vi "Car Wash.vi"() -> ()   [LabVIEW 2013]
uses:
  Controls/Car Wash Indicators.ctl
  Controls/Wash Options.ctl
  Controls/Car Wash States.ctl
  Controls/Wash option states.ctl
panel:
  in  "Start":bool
  out "Elapsed Time":dbl format="%0.2f"
  in  "stop":bool
  out "Wash Entry":bool
  in  "Wash Options":T1
  in  "Car Position Slider":u8(slide) max=3 scale=0.0..4.0
  out "Car Wash Indicators":T2
  # "Entry Console"
  # "Car Wash Display"
  # "Car Position Simulation"
  # "Pre-Soak\nH-P Wash\nL-P Wax\nSpot Free Rinse"
  # "Underbody Wash\nBug Remover"
  # "Tire Shine\nAir Dry"
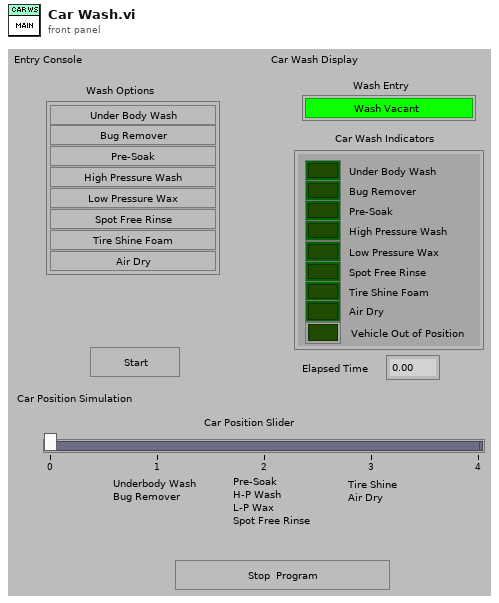
[diagram p1: front panel]
types:
  T1 = typedef "Wash Options.ctl" = cluster{"Underbody Wash":bool, "Bug Remover":bool, "Pre-Soak":bool, "High Pressure Wash":bool, "Low Pressure Wax":bool, "Spot Free Rinse":bool, "Tire Shine Foam":bool, "Air Dry":bool}
  T2 = typedef "Car Wash Indicators.ctl" = cluster{"Under Body Wash":bool, "Bug Remover":bool, "Pre-Soak":bool, "High Pressure Wash":bool, "Low Pressure Wax":bool, "Spot Free Rinse":bool, "Tire Shine Foam":bool, "Air Dry":bool, "Vehicle Out of Position":bool}
  T3 = typedef "Car Wash States.ctl" = enum16{"Initialize", "Start", "Main", "Stop"}
  T4 = enum8{"Enabled", "Disabled", "Disabled and Grayed Out"}
  T5 = typedef "Wash option states.ctl" = enum16{"Under Body Wash", "Bug Remover", "Pre-Soak", "HIgh Pressure Wash", "Low Pessure Wax", "Spot Free rinse", "Tire Shine Foam", "Air Dry", "Exit", "Reset "}
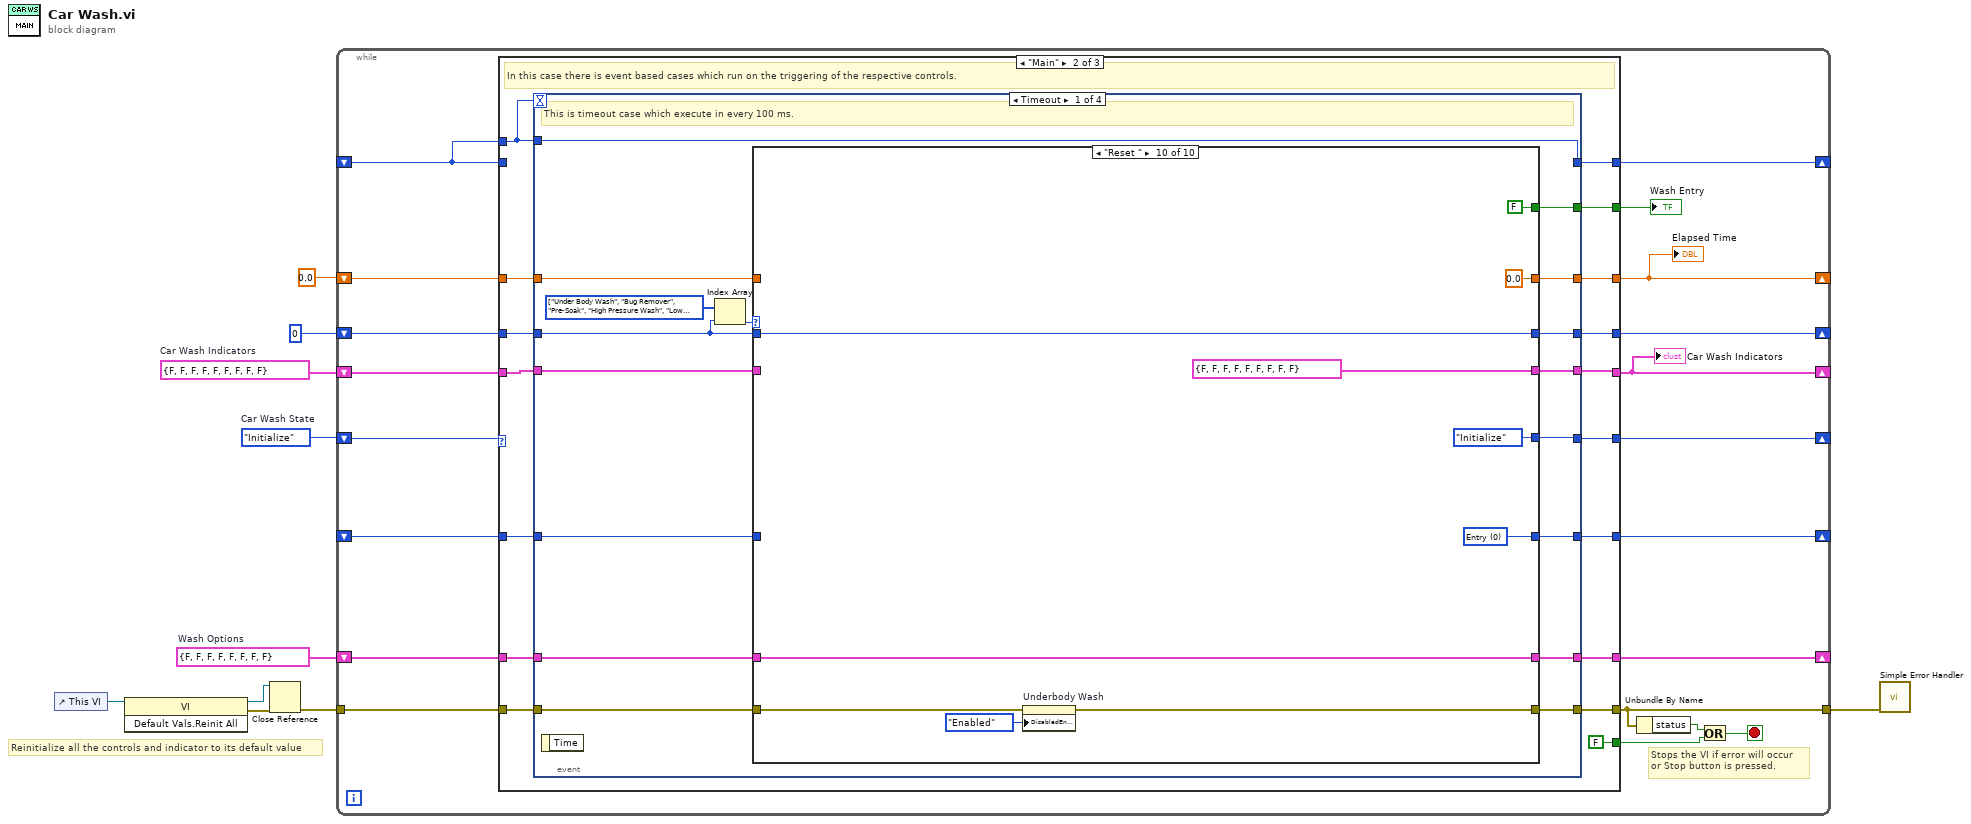
[diagram p0: block diagram]
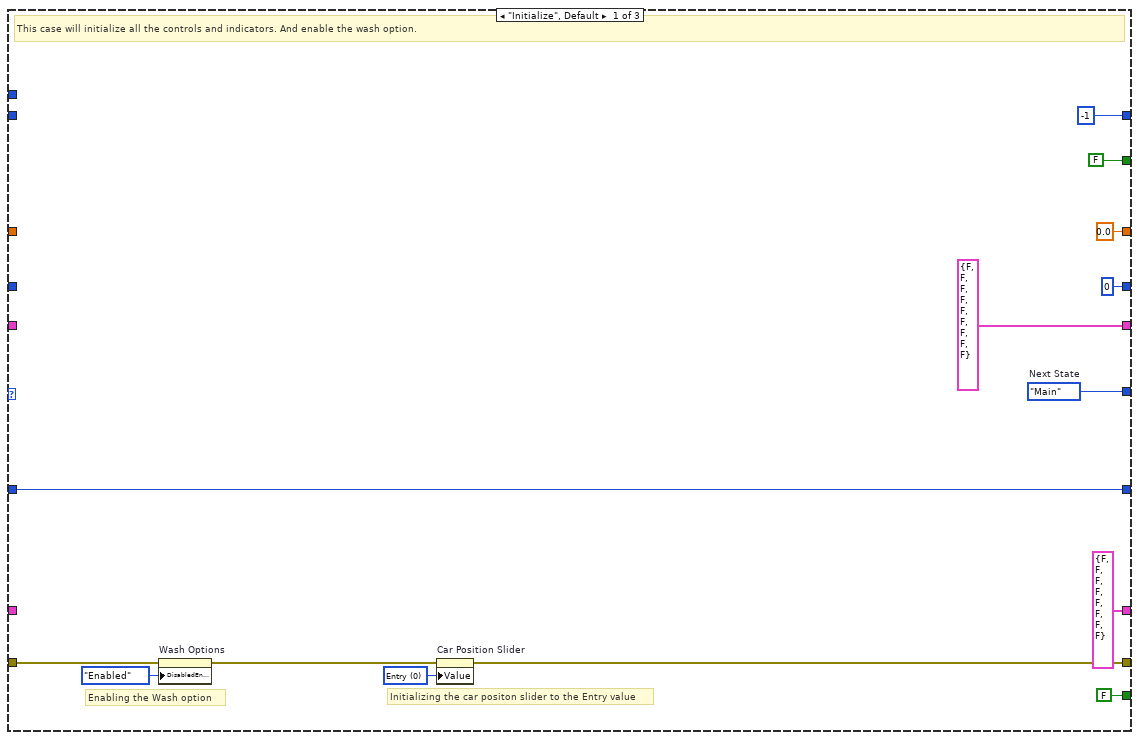
[diagram p2: hidden frame]
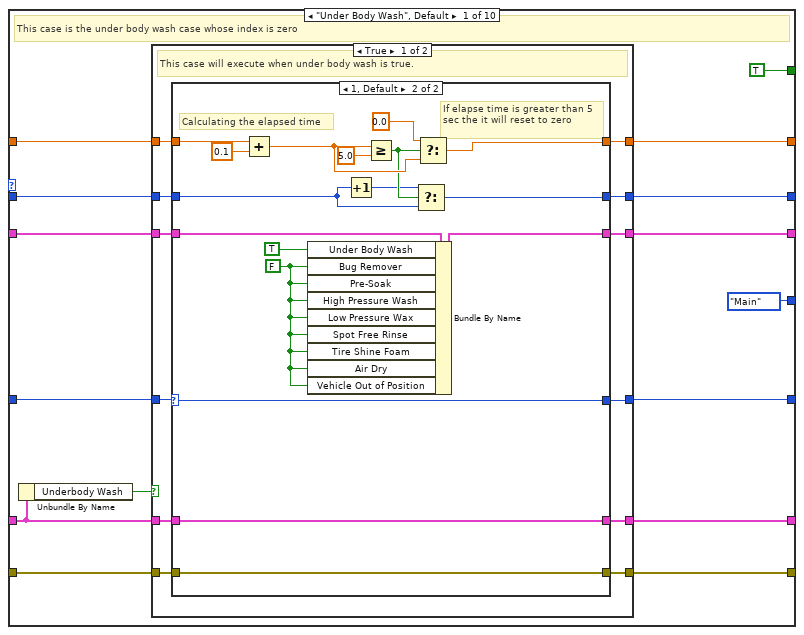
[diagram p3: hidden frame]
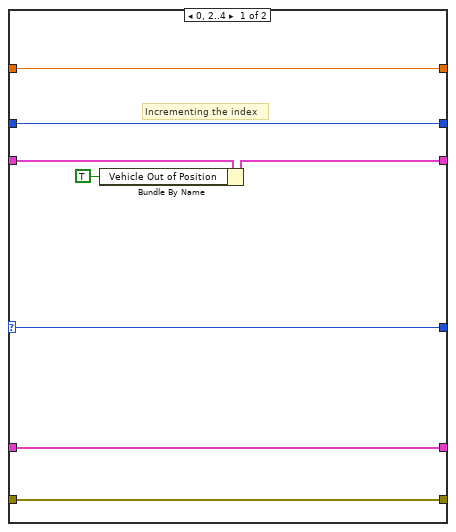
[diagram p4: hidden frame]
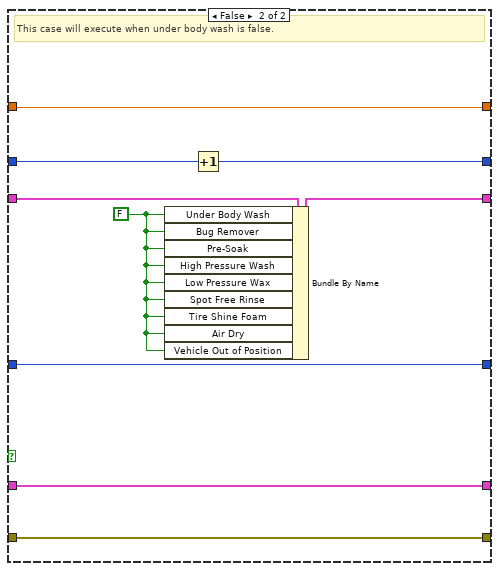
[diagram p5: hidden frame]
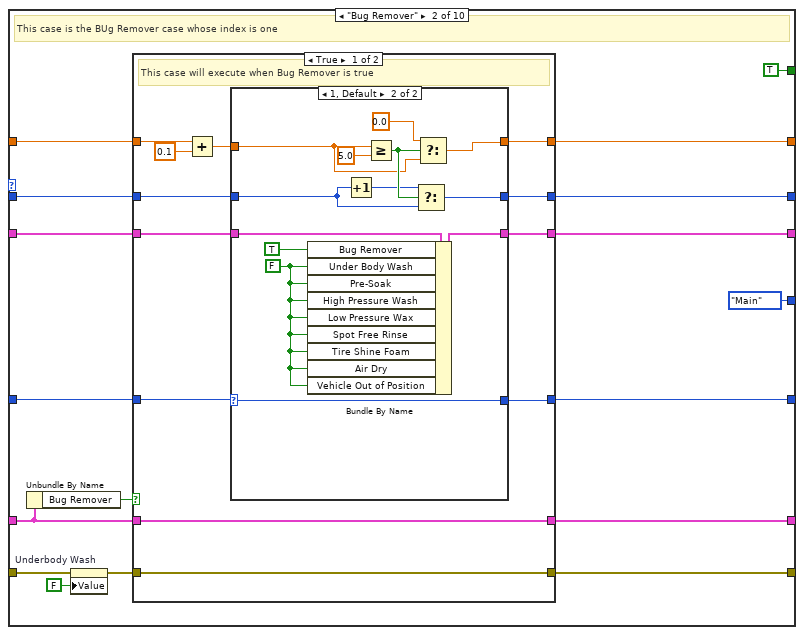
[diagram p6: hidden frame]
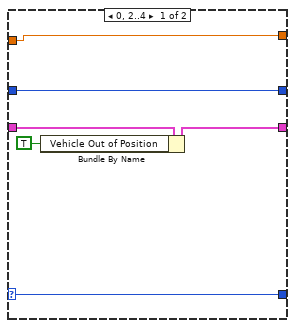
[diagram p7: hidden frame]
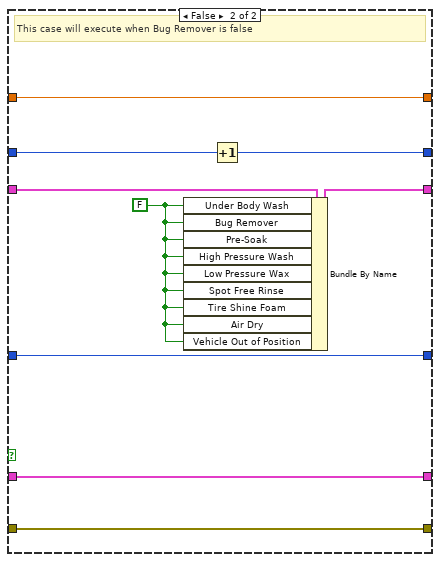
[diagram p8: hidden frame]
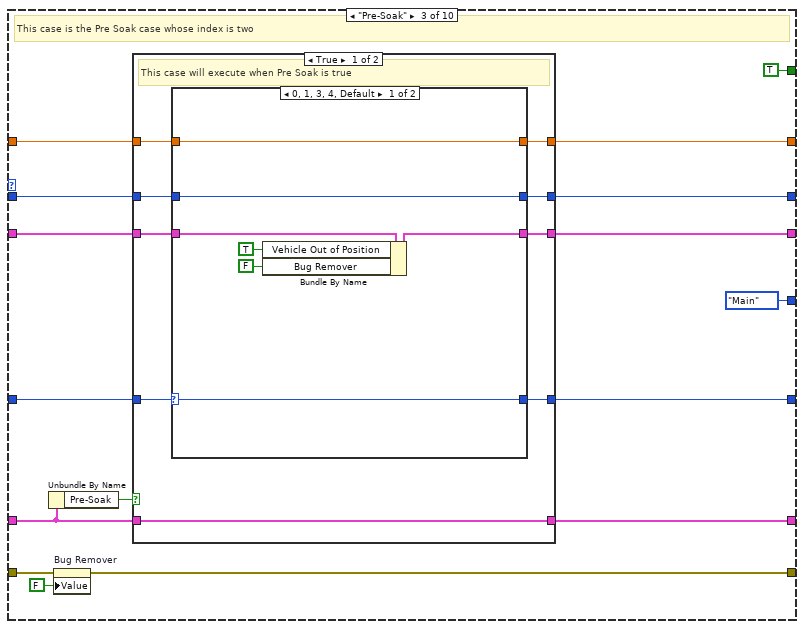
[diagram p9: hidden frame]
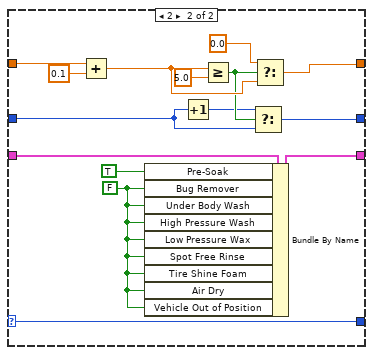
[diagram p10: hidden frame]
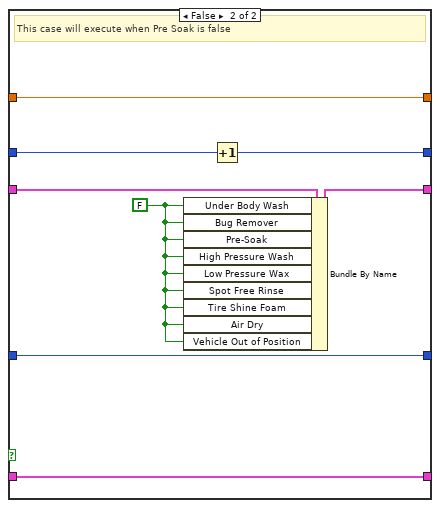
[diagram p11: hidden frame]
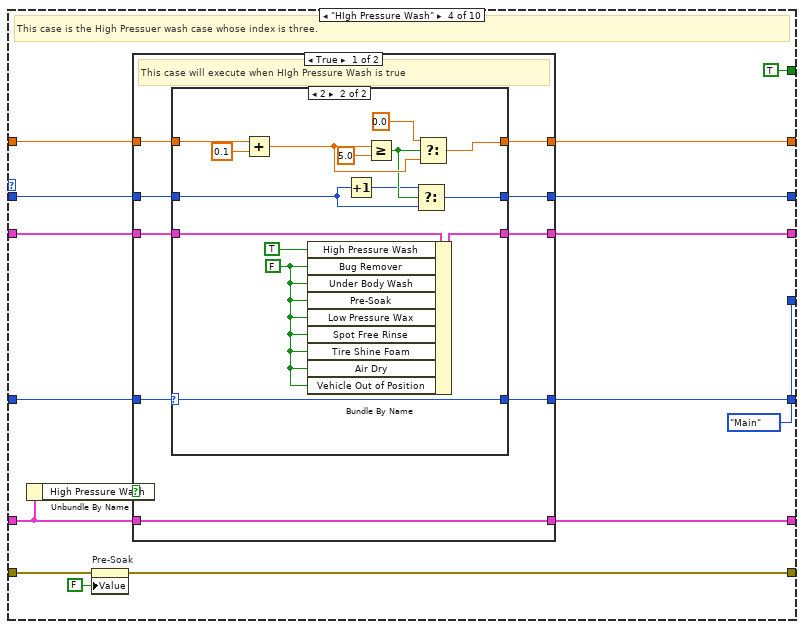
[diagram p12: hidden frame]
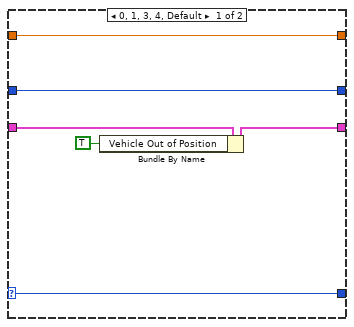
[diagram p13: hidden frame]
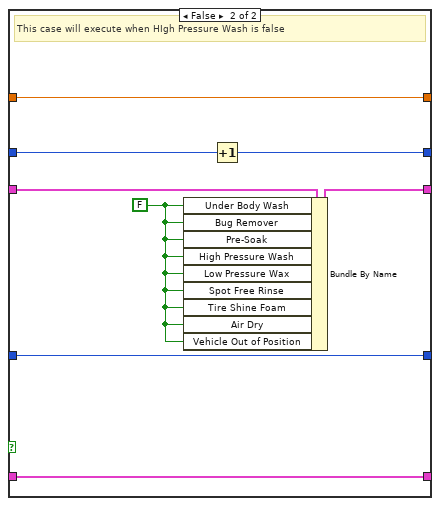
[diagram p14: hidden frame]
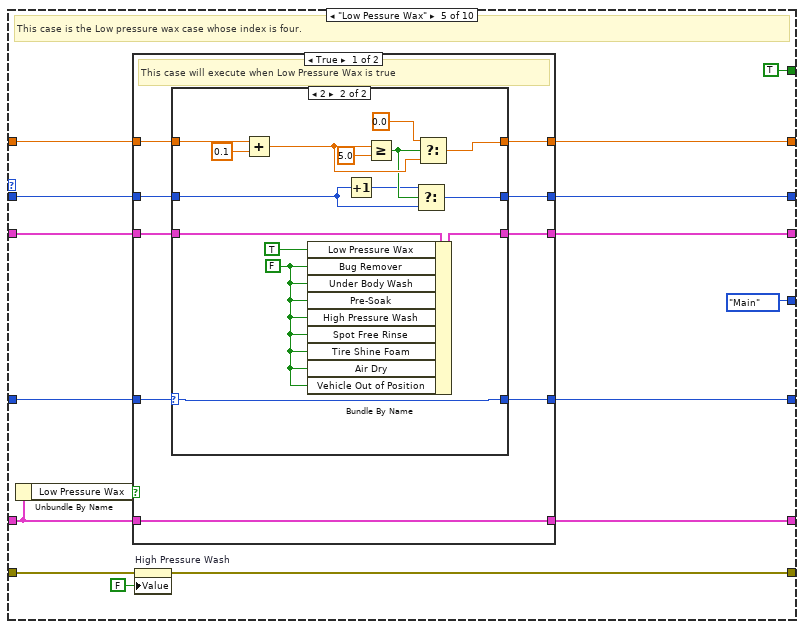
[diagram p15: hidden frame]
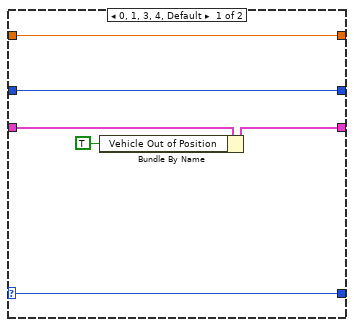
[diagram p16: hidden frame]
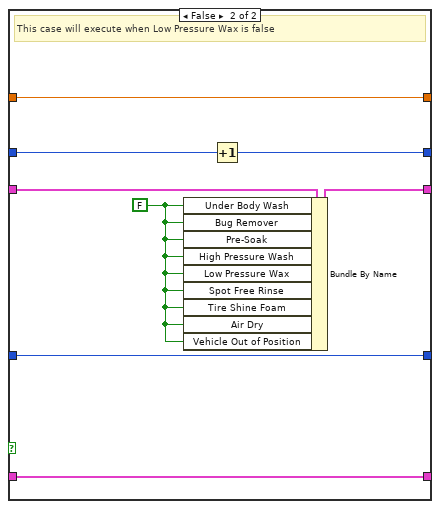
[diagram p17: hidden frame]
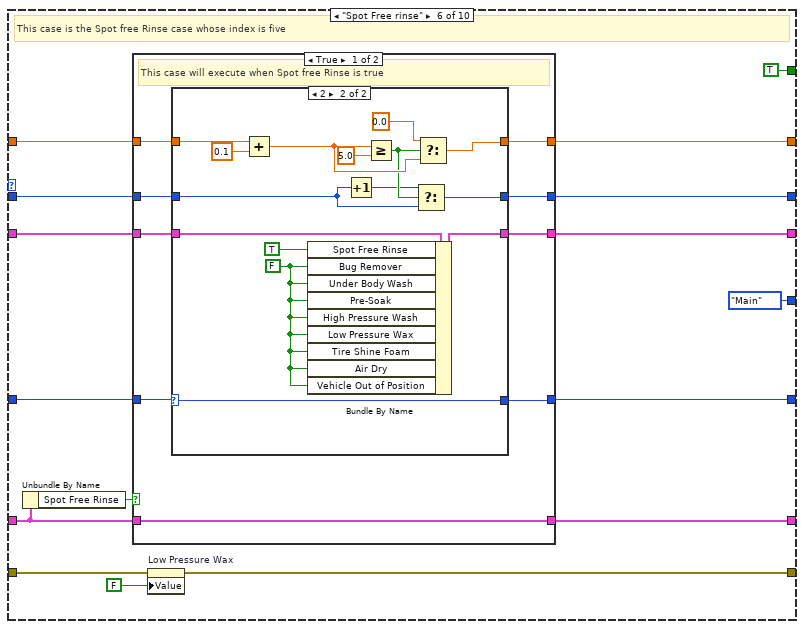
[diagram p18: hidden frame]
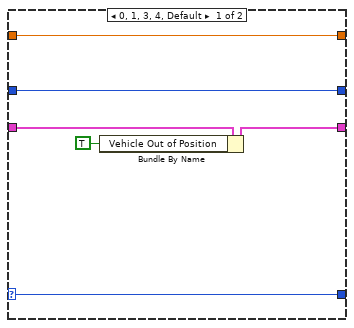
[diagram p19: hidden frame]
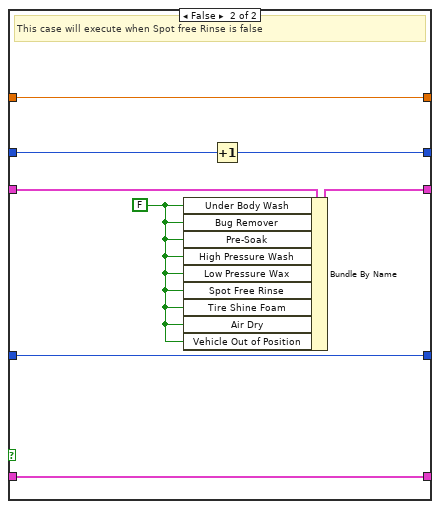
[diagram p20: hidden frame]
diagram:
  w2 = T2 {"Under Body Wash"=FALSE, "Bug Remover"=FALSE, "Pre-Soak"=FALSE, "High Pressure Wash"=FALSE, "Low Pressure Wax"=FALSE, "Spot Free Rinse"=FALSE, "Tire Shine Foam"=FALSE, "Air Dry"=FALSE, "Vehicle Out of Position"=FALSE}  # Car Wash Indicators
  w3 = T1 {"Underbody Wash"=FALSE, "Bug Remover"=FALSE, "Pre-Soak"=FALSE, "High Pressure Wash"=FALSE, "Low Pressure Wax"=FALSE, "Spot Free Rinse"=FALSE, "Tire Shine Foam"=FALSE, "Air Dry"=FALSE}  # Wash Options
  w10 = Car_Wash_States."Initialize"  # Car Wash State
  # "Reinitialize all the controls and indicator to its default value"
  n1 = control-ref of="This VI"() -> (w9:refnum<vi>)
  n2 = invoke class="VI" method="Default Vals.Reinit All"(reference=w9) -> (reference out=w7:refnum<vi>, error out=w8:errorcluster)  [unwired: 2 in, 1 out]
  n3 = Close Reference(reference=w7, error in (no error)=w8) -> (error out=w6:errorcluster)
  n4 = while {
    shift-right: [w29] -> _
    shift-left: w10 -> [w30]
    tunnel: w6 -> [w28]
    tunnel: [w23] -> w5
    shift-right: [w27] -> _
    shift-left: _ -> [w25]
    shift-right: [w15] -> _
    shift-left: 0.0 -> [w26]
    shift-right: [w19] -> _
    shift-left: w3 -> [w18]
    shift-right: [w17] -> _
    shift-left: _ -> [w16]
    shift-right: [w12] -> _
    shift-left: 0 -> [w13]
    shift-right: [w11] -> _
    shift-left: w2 -> [w14]
    stop <- w20 stop-if-true
    # "Stops the VI if error will occur \nor Stop button is pressed."
    n5 = case shown="\"Main\"" w30 {
      tunnel: [w44 w59 Car_Wash_States."Stop" ("Next State")] -> w29
      tunnel: w28 -> [w41 w60 w611]
      tunnel: [w40 w61 w608] -> w23
      tunnel: [-1 w50 0] -> w27
      tunnel: w25 -> [_ w49 _]
      tunnel: [0.0 ("t") w58 0.0 ("t")] -> w15
      tunnel: w26 -> [_ w57 _]
      tunnel: w25 -> [_ _ _]
      tunnel: [FALSE w46 FALSE] -> w24
      tunnel: [FALSE FALSE TRUE] -> w21
      tunnel: [T1 {"Underbody Wash"=FALSE, "Bug Remover"=FALSE, "Pre-Soak"=FALSE, "High Pressure Wash"=FALSE, "Low Pressure Wax"=FALSE, "Spot Free Rinse"=FALSE, "Tire Shine Foam"=FALSE, "Air Dry"=FALSE} ("Wash Options") w45 w616] -> w19
      tunnel: w18 -> [_ w55 w616]
      tunnel: [w34 w54 w612] -> w17
      tunnel: w16 -> [w34 w53 _]
      tunnel: [T2 {"Under Body Wash"=FALSE, "Bug Remover"=FALSE, "Pre-Soak"=FALSE, "High Pressure Wash"=FALSE, "Low Pressure Wax"=FALSE, "Spot Free Rinse"=FALSE, "Tire Shine Foam"=FALSE, "Air Dry"=FALSE, "Vehicle Out of Position"=FALSE} ("Car Wash Indicators") w52 T2 {"Under Body Wash"=FALSE, "Bug Remover"=FALSE, "Pre-Soak"=FALSE, "High Pressure Wash"=FALSE, "Low Pressure Wax"=FALSE, "Spot Free Rinse"=FALSE, "Tire Shine Foam"=FALSE, "Air Dry"=FALSE, "Vehicle Out of Position"=FALSE} ("Car Wash Indicators")] -> w11
      tunnel: w14 -> [_ w51 _]
      tunnel: w13 -> [_ w48 _]
      tunnel: [0 w47 0] -> w12
      frame "Initialize", Default {
        w38 = u8 0 items=["Entry", "Station 1", "Station 2", "Station 3", "Exit"] ("Car Position Slider")
        w44 = Car_Wash_States."Main"  # Next State
        # "Enabling the Wash option"
        # "Initializing the car positon slider to the Entry value"
        # "This case will initialize all the controls and indicators. And enable the wash option."
        n6 = property on="Wash Options" class="Clust (strict)"(error in=w41, "DisabledEnum"=T4."Enabled" ("Disabled")) -> (error out=w42:errorcluster)  [unwired: 1 in, 1 out]
        n7 = property on="Car Position Slider" class="Slide (strict)"(error in=w42, "Value"=w38) -> (error out=w40:errorcluster)  [unwired: 1 in, 1 out]
      }
      frame "Main" {
        # "In this case there is event based cases which run on the triggering of the respective controls."
        n8 = event shown="[0] Timeout" {
          selector: _ -> [_ _ _ _]
          dyn-events: _ -> [_ _ _ _]
          timeout: w49 -> [_ _ _ _]
          tunnel: [w65 w577 w591 w603] -> w61
          tunnel: w60 -> [w66 w579 w591 w604]
          tunnel: [w64 Car_Wash_States."Main" ("Car Wash State") Car_Wash_States."Main" ("Car Wash State") Car_Wash_States."Stop" ("Car Wash State")] -> w59
          tunnel: [w75 0.0 ("t") w590 w599] -> w58
          tunnel: w57 -> [w74 _ w590 w599]
          tunnel: w55 -> [w76 _ w586 _]
          tunnel: [w67 w582 "Car Position Slider" u8 0 ("Car Position Slider")] -> w54
          tunnel: w53 -> [w68 w582 _ _]
          tunnel: [w73 T2 {"Under Body Wash"=FALSE, "Bug Remover"=FALSE, "Pre-Soak"=FALSE, "High Pressure Wash"=FALSE, "Low Pressure Wax"=FALSE, "Spot Free Rinse"=FALSE, "Tire Shine Foam"=FALSE, "Air Dry"=FALSE, "Vehicle Out of Position"=FALSE} ("Car Wash Indicators") w588 T2 {"Under Body Wash"=FALSE, "Bug Remover"=FALSE, "Pre-Soak"=FALSE, "High Pressure Wash"=FALSE, "Low Pressure Wax"=FALSE, "Spot Free Rinse"=FALSE, "Tire Shine Foam"=FALSE, "Air Dry"=FALSE, "Vehicle Out of Position"=FALSE} ("Car Wash Indicators")] -> w52
          tunnel: w51 -> [w72 _ w588 _]
          tunnel: [w71 100 w593 w601] -> w50
          tunnel: w49 -> [w71 _ w593 w601]
          tunnel: w48 -> [w69 _ w587 _]
          tunnel: [w70 0 w587 0] -> w47
          tunnel: [w63 FALSE TRUE FALSE] -> w46
          tunnel: [w62 w571 w586 T1 {"Underbody Wash"=FALSE, "Bug Remover"=FALSE, "Pre-Soak"=FALSE, "High Pressure Wash"=FALSE, "Low Pressure Wax"=FALSE, "Spot Free Rinse"=FALSE, "Tire Shine Foam"=FALSE, "Air Dry"=FALSE} ("Wash Options")] -> w45
          event Timeout {
            w78 = T5[] [enum."Under Body Wash", enum."Bug Remover", enum."Pre-Soak", enum."HIgh Pressure Wash", enum."Low Pessure Wax", enum."Spot Free rinse", enum."Tire Shine Foam", enum."Air Dry", enum."Exit", enum."Reset "] items=["Under Body Wash", "Bug Remover", "Pre-Soak", "HIgh Pressure Wash", "Low Pessure Wax", "Spot Free rinse", "Tire Shine Foam", "Air Dry", "Exit", "Reset "]
            # "This is timeout case which execute in every 100 ms."
            n9 = event-data() -> ()  [unwired: 1 in, 1 out]
            n10 = Index Array(array=w78, index=w69) -> (element=w77:T5)
            n11 = case shown="\"Reset \"" w77 {
              tunnel: w76 -> [w85 w148 w204 w259 w313 w367 w421 w476 w529 w565]
              tunnel: [w92 w155 w211 w266 w320 w374 w428 w483 w538 0.0 ("t")] -> w75
              tunnel: w74 -> [w91 w154 w210 w265 w319 w373 w427 w482 w537 _]
              tunnel: [w90 w153 w209 w264 w318 w372 w426 w481 w536 T2 {"Under Body Wash"=FALSE, "Bug Remover"=FALSE, "Pre-Soak"=FALSE, "High Pressure Wash"=FALSE, "Low Pressure Wax"=FALSE, "Spot Free Rinse"=FALSE, "Tire Shine Foam"=FALSE, "Air Dry"=FALSE, "Vehicle Out of Position"=FALSE} ("Car Wash Indicators")] -> w73
              tunnel: w72 -> [w89 w152 w208 w263 w317 w371 w425 w480 w535 _]
              tunnel: [w88 w151 w207 w262 w316 w370 w424 w479 w524 w569] -> w70
              tunnel: w69 -> [w87 w150 w206 w261 w315 w369 w423 w478 w523 w569]
              tunnel: [w86 w149 w205 w260 w314 w368 w422 w477 w530 w565] -> w62
              tunnel: w68 -> [w84 w147 w197 w258 w312 w366 w420 w475 w534 _]
              tunnel: [w83 w146 w203 w257 w311 w365 w419 w474 w533 w567] -> w67
              tunnel: w66 -> [w82 w145 w202 w256 w310 w364 w418 w473 w532 w563]
              tunnel: [w81 w141 w201 w255 w309 w363 w417 w472 w528 w562] -> w65
              tunnel: [Car_Wash_States."Main" ("Car Wash State") Car_Wash_States."Main" ("Car Wash State") Car_Wash_States."Main" ("Car Wash State") Car_Wash_States."Main" ("Car Wash State") Car_Wash_States."Main" ("Car Wash State") Car_Wash_States."Main" ("Car Wash State") Car_Wash_States."Main" ("Car Wash State") Car_Wash_States."Main" ("Car Wash State") w526 Car_Wash_States."Initialize" ("Car Wash State")] -> w64
              tunnel: [TRUE TRUE TRUE TRUE TRUE TRUE TRUE TRUE w525 FALSE] -> w63
              frame "Under Body Wash", Default {
                # "This case is the under body wash case whose index is zero"
                n12 = Unbundle By Name(w85) -> ("Underbody Wash"=w93:bool)
                n13 = case shown="True" w93 {
                  tunnel: [w105 w139] -> w92
                  tunnel: w91 -> [w104 w139]
                  tunnel: [w102 w137] -> w90
                  tunnel: w89 -> [w103 w138]
                  tunnel: [w100 w134] -> w88
                  tunnel: w87 -> [w101 w135]
                  tunnel: [w95 w136] -> w86
                  tunnel: w85 -> [w94 w136]
                  tunnel: w84 -> [w99 w132]
                  tunnel: [w98 w132] -> w83
                  tunnel: w82 -> [w96 w131]
                  tunnel: [w97 w131] -> w81
                  frame True {
                    # "This case will execute when under body wash is true."
                    n14 = case shown="1, Default" w99 {
                      selector: w99 -> [w108 w116]
                      tunnel: [w113 w126] -> w105
                      tunnel: w104 -> [w113 w125]
                      tunnel: w103 -> [w111 w124]
                      tunnel: [w110 w123] -> w102
                      tunnel: w101 -> [w112 w120]
                      tunnel: [w112 w119] -> w100
                      tunnel: [w108 w116] -> w98
                      tunnel: [w106 w115] -> w97
                      tunnel: w96 -> [w106 w115]
                      tunnel: [w107 w114] -> w95
                      tunnel: w94 -> [w107 w114]
                      frame 0, 2..4 {
                        # "Incrementing the index"
                        n15 = Bundle By Name(cluster=w111, "Vehicle Out of Position"=TRUE) -> (w110:T2)
                      }
                      frame 1, Default {
                        w117 = FALSE ("Bug Remover")
                        # "If elapse time is greater than 5 sec the it will reset to zero"
                        # "Calculating the elapsed time"
                        n16 = Add(x=w125, y=0.1) -> (x+y=w128:dbl)
                        n17 = Bundle By Name(cluster=w124, "Under Body Wash"=TRUE, "Bug Remover"=w117, "Pre-Soak"=w117, "High Pressure Wash"=w117, "Low Pressure Wax"=w117, "Spot Free Rinse"=w117, "Tire Shine Foam"=w117, "Air Dry"=w117, "Vehicle Out of Position"=w117) -> (w123:T2)
                        n18 = Increment(x=w120) -> (x+1=w118:i32)
                        n19 = Greater Or Equal?(x=w128, y=5.0) -> (x >= y?=w121:bool)
                        n20 = Select(t=w118, s=w121, f=w120) -> (s? t:f=w119:i32)
                        n21 = Select(t=0.0, s=w121, f=w128) -> (s? t:f=w126:dbl)
                      }
                    }
                  }
                  frame False {
                    w133 = FALSE ("Under Body Wash")
                    # "This case will execute when under body wash is false."
                    n22 = Bundle By Name(cluster=w138, "Under Body Wash"=w133, "Bug Remover"=w133, "Pre-Soak"=w133, "High Pressure Wash"=w133, "Low Pressure Wax"=w133, "Spot Free Rinse"=w133, "Tire Shine Foam"=w133, "Air Dry"=w133, "Vehicle Out of Position"=w133) -> (w137:T2)
                    n23 = Increment(x=w135) -> (x+1=w134:i32)
                  }
                }
              }
              frame "Bug Remover" {
                # "This case is the BUg Remover case whose index is one"
                n24 = Unbundle By Name(w148) -> ("Bug Remover"=w156:bool)
                n25 = property on="Underbody Wash" class="Bool (strict)"(error in=w145, "Value"=FALSE) -> (error out=w140:errorcluster)  [unwired: 1 in, 1 out]
                n26 = case shown="True" w156 {
                  tunnel: [w168 w196] -> w155
                  tunnel: w154 -> [w157 w196]
                  tunnel: [w166 w194] -> w153
                  tunnel: w152 -> [w167 w195]
                  tunnel: [w164 w191] -> w151
                  tunnel: w150 -> [w165 w192]
                  tunnel: [w163 w193] -> w149
                  tunnel: w148 -> [w163 w193]
                  tunnel: w147 -> [w162 w189]
                  tunnel: [w161 w189] -> w146
                  tunnel: [w160 w188] -> w141
                  tunnel: w140 -> [w160 w188]
                  frame True {
                    # "This case will execute when Bug Remover is true"
                    n27 = Add(x=w157, y=0.1) -> (x+y=w158:dbl)
                    n28 = case shown="1, Default" w162 {
                      selector: w162 -> [w170 w176]
                      tunnel: [w169 w185] -> w168
                      tunnel: w158 -> [w169 w175]
                      tunnel: w167 -> [w173 w184]
                      tunnel: [w172 w183] -> w166
                      tunnel: w165 -> [w174 w180]
                      tunnel: [w174 w179] -> w164
                      tunnel: [w170 w176] -> w161
                      frame 0, 2..4 {
                        n29 = Bundle By Name(cluster=w173, "Vehicle Out of Position"=TRUE) -> (w172:T2)
                      }
                      frame 1, Default {
                        w177 = FALSE ("Bug Remover")
                        n30 = Bundle By Name(cluster=w184, "Bug Remover"=TRUE ("Under Body Wash"), "Under Body Wash"=w177, "Pre-Soak"=w177, "High Pressure Wash"=w177, "Low Pressure Wax"=w177, "Spot Free Rinse"=w177, "Tire Shine Foam"=w177, "Air Dry"=w177, "Vehicle Out of Position"=w177) -> (w183:T2)
                        n31 = Increment(x=w180) -> (x+1=w178:i32)
                        n32 = Greater Or Equal?(x=w175, y=5.0) -> (x >= y?=w181:bool)
                        n33 = Select(t=w178, s=w181, f=w180) -> (s? t:f=w179:i32)
                        n34 = Select(t=0.0, s=w181, f=w175) -> (s? t:f=w185:dbl)
                      }
                    }
                  }
                  frame False {
                    w190 = FALSE ("Under Body Wash")
                    # "This case will execute when Bug Remover is false"
                    n35 = Bundle By Name(cluster=w195, "Under Body Wash"=w190, "Bug Remover"=w190, "Pre-Soak"=w190, "High Pressure Wash"=w190, "Low Pressure Wax"=w190, "Spot Free Rinse"=w190, "Tire Shine Foam"=w190, "Air Dry"=w190, "Vehicle Out of Position"=w190) -> (w194:T2)
                    n36 = Increment(x=w192) -> (x+1=w191:i32)
                  }
                }
              }
              frame "Pre-Soak" {
                # "This case is the Pre Soak case whose index is two"
                n37 = Unbundle By Name(w204) -> ("Pre-Soak"=w212:bool)
                n38 = property on="Bug Remover" class="Bool (strict)"(error in=w202, "Value"=FALSE) -> (error out=w201:errorcluster)  [unwired: 1 in, 1 out]
                n39 = case shown="True" w212 {
                  tunnel: [w221 w251] -> w211
                  tunnel: w210 -> [w220 w251]
                  tunnel: [w218 w249] -> w209
                  tunnel: w208 -> [w219 w250]
                  tunnel: [w216 w246] -> w207
                  tunnel: w206 -> [w217 w247]
                  tunnel: [w215 w248] -> w205
                  tunnel: w204 -> [w215 w248]
                  tunnel: w197 -> [w214 w244]
                  tunnel: [w213 w244] -> w203
                  frame True {
                    # "This case will execute when Pre Soak is true"
                    n40 = case shown="0, 1, 3, 4, Default" w214 {
                      selector: w214 -> [w223 w229]
                      tunnel: [w228 w239] -> w221
                      tunnel: w220 -> [w228 w238]
                      tunnel: w219 -> [w226 w237]
                      tunnel: [w225 w236] -> w218
                      tunnel: w217 -> [w227 w233]
                      tunnel: [w227 w232] -> w216
                      tunnel: [w223 w229] -> w213
                      frame 0, 1, 3, 4, Default {
                        n41 = Bundle By Name(cluster=w226, "Vehicle Out of Position"=TRUE, "Bug Remover"=FALSE) -> (w225:T2)
                      }
                      frame 2 {
                        w230 = FALSE ("Bug Remover")
                        n42 = Add(x=w238, y=0.1) -> (x+y=w241:dbl)
                        n43 = Bundle By Name(cluster=w237, "Pre-Soak"=TRUE ("Under Body Wash"), "Bug Remover"=w230, "Under Body Wash"=w230, "High Pressure Wash"=w230, "Low Pressure Wax"=w230, "Spot Free Rinse"=w230, "Tire Shine Foam"=w230, "Air Dry"=w230, "Vehicle Out of Position"=w230) -> (w236:T2)
                        n44 = Increment(x=w233) -> (x+1=w231:i32)
                        n45 = Greater Or Equal?(x=w241, y=5.0) -> (x >= y?=w234:bool)
                        n46 = Select(t=w231, s=w234, f=w233) -> (s? t:f=w232:i32)
                        n47 = Select(t=0.0, s=w234, f=w241) -> (s? t:f=w239:dbl)
                      }
                    }
                  }
                  frame False {
                    w245 = FALSE ("Under Body Wash")
                    # "This case will execute when Pre Soak is false"
                    n48 = Bundle By Name(cluster=w250, "Under Body Wash"=w245, "Bug Remover"=w245, "Pre-Soak"=w245, "High Pressure Wash"=w245, "Low Pressure Wax"=w245, "Spot Free Rinse"=w245, "Tire Shine Foam"=w245, "Air Dry"=w245, "Vehicle Out of Position"=w245) -> (w249:T2)
                    n49 = Increment(x=w247) -> (x+1=w246:i32)
                  }
                }
              }
              frame "HIgh Pressure Wash" {
                # "This case is the High Pressuer wash case whose index is three."
                n50 = Unbundle By Name(w259) -> ("High Pressure Wash"=w267:bool)
                n51 = property on="Pre-Soak" class="Bool (strict)"(error in=w256, "Value"=FALSE) -> (error out=w255:errorcluster)  [unwired: 1 in, 1 out]
                n52 = case shown="True" w267 {
                  tunnel: [w276 w305] -> w266
                  tunnel: w265 -> [w275 w305]
                  tunnel: [w273 w303] -> w264
                  tunnel: w263 -> [w274 w304]
                  tunnel: [w271 w300] -> w262
                  tunnel: w261 -> [w272 w301]
                  tunnel: [w270 w302] -> w260
                  tunnel: w259 -> [w270 w302]
                  tunnel: w258 -> [w269 w298]
                  tunnel: [w268 w298] -> w257
                  frame True {
                    # "This case will execute when HIgh Pressure Wash is true"
                    n53 = case shown="2" w269 {
                      selector: w269 -> [w277 w283]
                      tunnel: [w282 w293] -> w276
                      tunnel: w275 -> [w282 w292]
                      tunnel: w274 -> [w280 w291]
                      tunnel: [w279 w290] -> w273
                      tunnel: w272 -> [w281 w287]
                      tunnel: [w281 w286] -> w271
                      tunnel: [w277 w283] -> w268
                      frame 0, 1, 3, 4, Default {
                        n54 = Bundle By Name(cluster=w280, "Vehicle Out of Position"=TRUE) -> (w279:T2)
                      }
                      frame 2 {
                        w284 = FALSE ("Bug Remover")
                        n55 = Add(x=w292, y=0.1) -> (x+y=w295:dbl)
                        n56 = Bundle By Name(cluster=w291, "High Pressure Wash"=TRUE ("Under Body Wash"), "Bug Remover"=w284, "Under Body Wash"=w284, "Pre-Soak"=w284, "Low Pressure Wax"=w284, "Spot Free Rinse"=w284, "Tire Shine Foam"=w284, "Air Dry"=w284, "Vehicle Out of Position"=w284) -> (w290:T2)
                        n57 = Increment(x=w287) -> (x+1=w285:i32)
                        n58 = Greater Or Equal?(x=w295, y=5.0) -> (x >= y?=w288:bool)
                        n59 = Select(t=w285, s=w288, f=w287) -> (s? t:f=w286:i32)
                        n60 = Select(t=0.0, s=w288, f=w295) -> (s? t:f=w293:dbl)
                      }
                    }
                  }
                  frame False {
                    w299 = FALSE ("Under Body Wash")
                    # "This case will execute when HIgh Pressure Wash is false"
                    n61 = Bundle By Name(cluster=w304, "Under Body Wash"=w299, "Bug Remover"=w299, "Pre-Soak"=w299, "High Pressure Wash"=w299, "Low Pressure Wax"=w299, "Spot Free Rinse"=w299, "Tire Shine Foam"=w299, "Air Dry"=w299, "Vehicle Out of Position"=w299) -> (w303:T2)
                    n62 = Increment(x=w301) -> (x+1=w300:i32)
                  }
                }
              }
              frame "Low Pessure Wax" {
                # "This case is the Low pressure wax case whose index is four."
                n63 = Unbundle By Name(w313) -> ("Low Pressure Wax"=w321:bool)
                n64 = case shown="True" w321 {
                  tunnel: [w330 w359] -> w320
                  tunnel: w319 -> [w329 w359]
                  tunnel: [w327 w357] -> w318
                  tunnel: w317 -> [w328 w358]
                  tunnel: [w325 w354] -> w316
                  tunnel: w315 -> [w326 w355]
                  tunnel: [w324 w356] -> w314
                  tunnel: w313 -> [w324 w356]
                  tunnel: w312 -> [w323 w352]
                  tunnel: [w322 w352] -> w311
                  frame True {
                    # "This case will execute when Low Pressure Wax is true"
                    n65 = case shown="2" w323 {
                      selector: w323 -> [w331 w337]
                      tunnel: [w336 w347] -> w330
                      tunnel: w329 -> [w336 w346]
                      tunnel: w328 -> [w334 w345]
                      tunnel: [w333 w344] -> w327
                      tunnel: w326 -> [w335 w341]
                      tunnel: [w335 w340] -> w325
                      tunnel: [w331 w337] -> w322
                      frame 0, 1, 3, 4, Default {
                        n66 = Bundle By Name(cluster=w334, "Vehicle Out of Position"=TRUE) -> (w333:T2)
                      }
                      frame 2 {
                        w338 = FALSE ("Bug Remover")
                        n67 = Add(x=w346, y=0.1) -> (x+y=w349:dbl)
                        n68 = Bundle By Name(cluster=w345, "Low Pressure Wax"=TRUE ("Under Body Wash"), "Bug Remover"=w338, "Under Body Wash"=w338, "Pre-Soak"=w338, "High Pressure Wash"=w338, "Spot Free Rinse"=w338, "Tire Shine Foam"=w338, "Air Dry"=w338, "Vehicle Out of Position"=w338) -> (w344:T2)
                        n69 = Increment(x=w341) -> (x+1=w339:i32)
                        n70 = Greater Or Equal?(x=w349, y=5.0) -> (x >= y?=w342:bool)
                        n71 = Select(t=w339, s=w342, f=w341) -> (s? t:f=w340:i32)
                        n72 = Select(t=0.0, s=w342, f=w349) -> (s? t:f=w347:dbl)
                      }
                    }
                  }
                  frame False {
                    w353 = FALSE ("Under Body Wash")
                    # "This case will execute when Low Pressure Wax is false"
                    n73 = Bundle By Name(cluster=w358, "Under Body Wash"=w353, "Bug Remover"=w353, "Pre-Soak"=w353, "High Pressure Wash"=w353, "Low Pressure Wax"=w353, "Spot Free Rinse"=w353, "Tire Shine Foam"=w353, "Air Dry"=w353, "Vehicle Out of Position"=w353) -> (w357:T2)
                    n74 = Increment(x=w355) -> (x+1=w354:i32)
                  }
                }
                n75 = property on="High Pressure Wash" class="Bool (strict)"(error in=w310, "Value"=FALSE) -> (error out=w309:errorcluster)  [unwired: 1 in, 1 out]
              }
              frame "Spot Free rinse" {
                # "This case is the Spot free Rinse case whose index is five"
                n76 = Unbundle By Name(w367) -> ("Spot Free Rinse"=w375:bool)
                n77 = case shown="True" w375 {
                  tunnel: [w384 w413] -> w374
                  tunnel: w373 -> [w383 w413]
                  tunnel: [w381 w411] -> w372
                  tunnel: w371 -> [w382 w412]
                  tunnel: [w379 w408] -> w370
                  tunnel: w369 -> [w380 w409]
                  tunnel: [w378 w410] -> w368
                  tunnel: w367 -> [w378 w410]
                  tunnel: w366 -> [w377 w406]
                  tunnel: [w376 w406] -> w365
                  frame True {
                    # "This case will execute when Spot free Rinse is true"
                    n78 = case shown="2" w377 {
                      selector: w377 -> [w385 w391]
                      tunnel: [w390 w401] -> w384
                      tunnel: w383 -> [w390 w400]
                      tunnel: w382 -> [w388 w399]
                      tunnel: [w387 w398] -> w381
                      tunnel: w380 -> [w389 w395]
                      tunnel: [w389 w394] -> w379
                      tunnel: [w385 w391] -> w376
                      frame 0, 1, 3, 4, Default {
                        n79 = Bundle By Name(cluster=w388, "Vehicle Out of Position"=TRUE) -> (w387:T2)
                      }
                      frame 2 {
                        w392 = FALSE ("Bug Remover")
                        n80 = Add(x=w400, y=0.1) -> (x+y=w403:dbl)
                        n81 = Bundle By Name(cluster=w399, "Spot Free Rinse"=TRUE ("Under Body Wash"), "Bug Remover"=w392, "Under Body Wash"=w392, "Pre-Soak"=w392, "High Pressure Wash"=w392, "Low Pressure Wax"=w392, "Tire Shine Foam"=w392, "Air Dry"=w392, "Vehicle Out of Position"=w392) -> (w398:T2)
                        n82 = Increment(x=w395) -> (x+1=w393:i32)
                        n83 = Greater Or Equal?(x=w403, y=5.0) -> (x >= y?=w396:bool)
                        n84 = Select(t=w393, s=w396, f=w395) -> (s? t:f=w394:i32)
                        n85 = Select(t=0.0, s=w396, f=w403) -> (s? t:f=w401:dbl)
                      }
                    }
                  }
                  frame False {
                    w407 = FALSE ("Under Body Wash")
                    # "This case will execute when Spot free Rinse is false"
                    n86 = Bundle By Name(cluster=w412, "Under Body Wash"=w407, "Bug Remover"=w407, "Pre-Soak"=w407, "High Pressure Wash"=w407, "Low Pressure Wax"=w407, "Spot Free Rinse"=w407, "Tire Shine Foam"=w407, "Air Dry"=w407, "Vehicle Out of Position"=w407) -> (w411:T2)
                    n87 = Increment(x=w409) -> (x+1=w408:i32)
                  }
                }
                n88 = property on="Low Pressure Wax" class="Bool (strict)"(error in=w364, "Value"=FALSE) -> (error out=w363:errorcluster)  [unwired: 1 in, 1 out]
              }
              frame "Tire Shine Foam" {
                # "This case is the Tire Shine Foam case whose index is six"
                n89 = Unbundle By Name(w421) -> ("Tire Shine Foam"=w429:bool)
                n90 = property on="Spot Free Rinse" class="Bool (strict)"(error in=w418, "Value"=FALSE) -> (error out=w417:errorcluster)  [unwired: 1 in, 1 out]
                n91 = case shown="True" w429 {
                  tunnel: [w438 w468] -> w428
                  tunnel: w427 -> [w437 w468]
                  tunnel: [w435 w466] -> w426
                  tunnel: w425 -> [w436 w467]
                  tunnel: [w433 w463] -> w424
                  tunnel: w423 -> [w434 w464]
                  tunnel: [w432 w465] -> w422
                  tunnel: w421 -> [w432 w465]
                  tunnel: w420 -> [w431 w461]
                  tunnel: [w430 w461] -> w419
                  frame True {
                    # "This case will execute when Tire Shine Foam is true"
                    n92 = case shown="0..2, 4, Default" w431 {
                      selector: w431 -> [w440 w446]
                      tunnel: [w445 w456] -> w438
                      tunnel: w437 -> [w445 w455]
                      tunnel: w436 -> [w443 w454]
                      tunnel: [w442 w453] -> w435
                      tunnel: w434 -> [w444 w450]
                      tunnel: [w444 w449] -> w433
                      tunnel: [w440 w446] -> w430
                      frame 0..2, 4, Default {
                        n93 = Bundle By Name(cluster=w443, "Vehicle Out of Position"=TRUE, "Spot Free Rinse"=FALSE) -> (w442:T2)
                      }
                      frame 3 {
                        w447 = FALSE ("Bug Remover")
                        n94 = Add(x=w455, y=0.1) -> (x+y=w458:dbl)
                        n95 = Bundle By Name(cluster=w454, "Tire Shine Foam"=TRUE ("Under Body Wash"), "Bug Remover"=w447, "Under Body Wash"=w447, "Pre-Soak"=w447, "High Pressure Wash"=w447, "Low Pressure Wax"=w447, "Spot Free Rinse"=w447, "Air Dry"=w447, "Vehicle Out of Position"=w447) -> (w453:T2)
                        n96 = Increment(x=w450) -> (x+1=w448:i32)
                        n97 = Greater Or Equal?(x=w458, y=5.0) -> (x >= y?=w451:bool)
                        n98 = Select(t=w448, s=w451, f=w450) -> (s? t:f=w449:i32)
                        n99 = Select(t=0.0, s=w451, f=w458) -> (s? t:f=w456:dbl)
                      }
                    }
                  }
                  frame False {
                    w462 = FALSE ("Under Body Wash")
                    # "This case will execute when Tire Shine Foam is true"
                    n100 = Bundle By Name(cluster=w467, "Under Body Wash"=w462, "Bug Remover"=w462, "Pre-Soak"=w462, "High Pressure Wash"=w462, "Low Pressure Wax"=w462, "Spot Free Rinse"=w462, "Tire Shine Foam"=w462, "Air Dry"=w462, "Vehicle Out of Position"=w462) -> (w466:T2)
                    n101 = Increment(x=w464) -> (x+1=w463:i32)
                  }
                }
              }
              frame "Air Dry" {
                # "This case is the Air Dry case whose index is seven."
                n102 = Unbundle By Name(w476) -> ("Air Dry"=w484:bool)
                n103 = case shown="True" w484 {
                  tunnel: [w493 w522] -> w483
                  tunnel: w482 -> [w492 w522]
                  tunnel: [w490 w520] -> w481
                  tunnel: w480 -> [w491 w521]
                  tunnel: [w488 w517] -> w479
                  tunnel: w478 -> [w489 w518]
                  tunnel: [w487 w519] -> w477
                  tunnel: w476 -> [w487 w519]
                  tunnel: w475 -> [w486 w515]
                  tunnel: [w485 w515] -> w474
                  frame True {
                    # "This case will execute when Air Dry is true"
                    n104 = case shown="3" w486 {
                      selector: w486 -> [w494 w500]
                      tunnel: [w499 w510] -> w493
                      tunnel: w492 -> [w499 w509]
                      tunnel: w491 -> [w497 w508]
                      tunnel: [w496 w507] -> w490
                      tunnel: w489 -> [w498 w504]
                      tunnel: [w498 w503] -> w488
                      tunnel: [w494 w500] -> w485
                      frame 0..2, 4, Default {
                        n105 = Bundle By Name(cluster=w497, "Vehicle Out of Position"=TRUE) -> (w496:T2)
                      }
                      frame 3 {
                        w501 = FALSE ("Bug Remover")
                        n106 = Add(x=w509, y=0.1) -> (x+y=w512:dbl)
                        n107 = Bundle By Name(cluster=w508, "Air Dry"=TRUE ("Under Body Wash"), "Bug Remover"=w501, "Under Body Wash"=w501, "Pre-Soak"=w501, "High Pressure Wash"=w501, "Low Pressure Wax"=w501, "Spot Free Rinse"=w501, "Tire Shine Foam"=w501, "Vehicle Out of Position"=w501) -> (w507:T2)
                        n108 = Increment(x=w504) -> (x+1=w502:i32)
                        n109 = Greater Or Equal?(x=w512, y=5.0) -> (x >= y?=w505:bool)
                        n110 = Select(t=w502, s=w505, f=w504) -> (s? t:f=w503:i32)
                        n111 = Select(t=0.0, s=w505, f=w512) -> (s? t:f=w510:dbl)
                      }
                    }
                  }
                  frame False {
                    w516 = FALSE ("Under Body Wash")
                    # "This case will execute when Air Dry is false"
                    n112 = Bundle By Name(cluster=w521, "Under Body Wash"=w516, "Bug Remover"=w516, "Pre-Soak"=w516, "High Pressure Wash"=w516, "Low Pressure Wax"=w516, "Spot Free Rinse"=w516, "Tire Shine Foam"=w516, "Air Dry"=w516, "Vehicle Out of Position"=w516) -> (w520:T2)
                    n113 = Increment(x=w518) -> (x+1=w517:i32)
                  }
                }
                n114 = property on="Tire Shine Foam" class="Bool (strict)"(error in=w473, "Value"=FALSE) -> (error out=w472:errorcluster)  [unwired: 1 in, 1 out]
              }
              frame "Exit" {
                n115 = property on="Air Dry" class="Bool (strict)"(error in=w532, "Value"=FALSE) -> (error out=w527:errorcluster)  [unwired: 1 in, 1 out]
                n116 = case shown="0..3, Default" w534 {
                  selector: w534 -> [w545 _]
                  tunnel: [w549 0.0 ("t")] -> w538
                  tunnel: w537 -> [w549 _]
                  tunnel: w535 -> [w548 w553]
                  tunnel: [w547 w553] -> w536
                  tunnel: [w545 w559] -> w533
                  tunnel: [w544 w557] -> w530
                  tunnel: w529 -> [w544 w557]
                  tunnel: [w543 w555] -> w528
                  tunnel: w527 -> [w543 w556]
                  tunnel: [Car_Wash_States."Main" ("Car Wash State") Car_Wash_States."Main" ("Car Wash State")] -> w526
                  tunnel: [TRUE FALSE] -> w525
                  tunnel: [w540 w550] -> w524
                  tunnel: w523 -> [w540 w551]
                  frame 0..3, Default {
                    n117 = Bundle By Name(cluster=w548, "Vehicle Out of Position"=TRUE, "Air Dry"=FALSE) -> (w547:T2)
                  }
                  frame 4 {
                    w558 = u8 0 items=["Entry", "Station 1", "Station 2", "Station 3", "Exit"] ("Car Position Slider")
                    w559 = u8 0 items=["Entry", "Station 1", "Station 2", "Station 3", "Exit"] ("Car Position Slider")
                    n118 = Increment(x=w551) -> (x+1=w550:i32)
                    n119 = property on="Car Position Slider" class="Slide (strict)"(error in=w556, "Value"=w558) -> (error out=w555:errorcluster)  [unwired: 1 in, 1 out]
                  }
                }
              }
              frame "Reset " {
                w567 = u8 0 items=["Entry", "Station 1", "Station 2", "Station 3", "Exit"] ("Car Position Slider")
                n120 = property on="Underbody Wash" class="Bool (strict)"(error in=w563, "DisabledEnum"=T4."Enabled" ("Disabled")) -> (error out=w562:errorcluster)  [unwired: 1 in, 1 out]
              }
            }
          }
          event "Start": Value Change {
            # "When Start button will pressed then this event will trigger. Which stores the value of wash option in shift register. And disable the Wash option.."
            n121 = event-data() -> ()  [unwired: 1 in, 2 out]
            n122 = property on="High Pressure Wash" class="Bool (strict)"(error in=w579, "Value"=TRUE) -> (error out=w578:errorcluster)  [unwired: 1 in, 1 out]
            n123 = property on="Wash Options" class="Clust (strict)"(error in=w578, "DisabledEnum"=T4."Disabled and Grayed Out" ("Disabled")) -> (error out=w577:errorcluster)  [unwired: 1 in, 1 out]
            n124 = Bundle By Name(cluster="Wash Options", "High Pressure Wash"=TRUE) -> (w571:T1)
          }
          event "Car Position Slider": Value Change {
            # "This event will pass the value of Car position slider."
            n125 = event-data() -> ()  [unwired: 1 in, 1 out]
          }
          event "stop": Value Change {
            # "This event will trigger the Stop case and stop the VI."
            n126 = event-data() -> ()  [unwired: 1 in, 6 out]
            n127 = property on="Wash Options" class="Clust (strict)"(error in=w604, "DisabledEnum"=T4."Disabled and Grayed Out" ("Disabled")) -> (error out=w603:errorcluster)  [unwired: 1 in, 1 out]
          }
        }
      }
      frame "Stop" {
        w607 = u8 0 items=["Entry", "Station 1", "Station 2", "Station 3", "Exit"] ("Car Position Slider")
        w612 = u8 0 items=["Entry", "Station 1", "Station 2", "Station 3", "Exit"] ("Car Position Slider")
        n128 = property on="Wash Options" class="Clust (strict)"(error in=w611, "Value"=T1 {"Underbody Wash"=FALSE, "Bug Remover"=FALSE, "Pre-Soak"=FALSE, "High Pressure Wash"=FALSE, "Low Pressure Wax"=FALSE, "Spot Free Rinse"=FALSE, "Tire Shine Foam"=FALSE, "Air Dry"=FALSE} ("Wash Options")) -> (error out=w609:errorcluster)  [unwired: 1 in, 1 out]
        n129 = property on="Car Position Slider" class="Slide (strict)"(error in=w609, "Value"=w607) -> (error out=w608:errorcluster)  [unwired: 1 in, 1 out]
      }
    }
    "Wash Entry" <- w24
    "Elapsed Time" <- w15
    "Car Wash Indicators" <- w11
    n130 = Unbundle By Name(w23) -> ("status"=w22:bool)
    n131 = Or(x=w22, y=w21) -> (x .or. y?=w20:bool)
  }
  n132 = call <vilib>:"Simple Error Handler.vi"("error in (no error)"=w5) -> ()  [unwired: 4 in, 5 out]
